vi "Open Data File.vi"(8 "error in (no error)":errorcluster, 11 "DbMeasurement in":refnum<class "DbMeasurement.lvclass">) -> (0 "error out":errorcluster, 3 "DbMeasurement out":refnum<class "DbMeasurement.lvclass">)   [LabVIEW 2013, in "DbMeasurement.lvclass"]
doc: "This static method opens the data file, which points to a database link."
uses:
  DbMeasurement.lvclass
  BaseMeasurement/BaseMeasurement.lvclass/BaseMeasurement.ctl
  DbMeasurement.lvclass/DbMeasurement.ctl
  <vilib>/addons/database/Connection.llb/DB Tools Open Connec (String).vi
  BaseMeasurement/BaseMeasurement.lvclass
  <vilib>/addons/database/NI_Database_API.lvlib
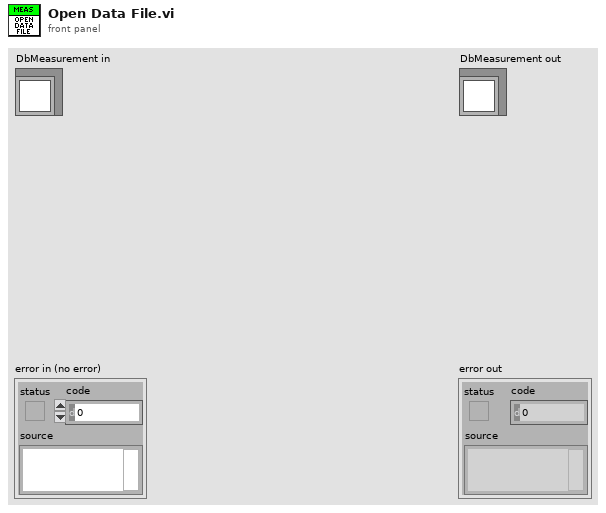
[diagram p1: front panel]
types:
  T1 = typedef "NI_Database_API.lvlib/Conn ObjectReference.ctl" = refnum<k1>
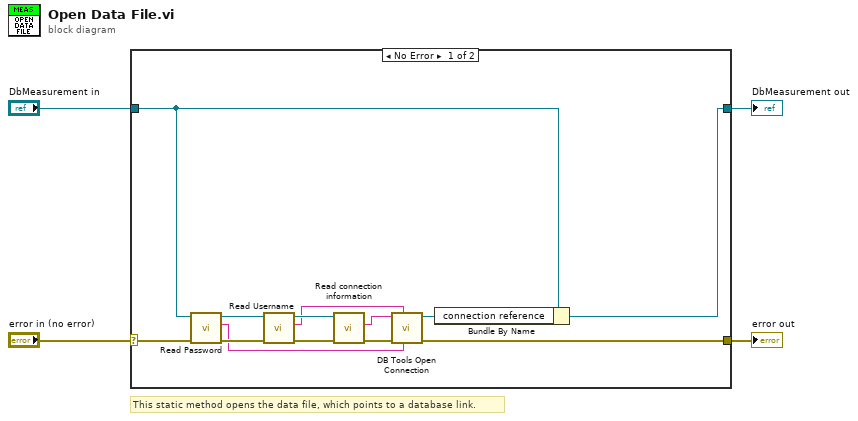
[diagram p0: block diagram]
diagram:
  # "This static method opens the data file, which points to a database link."
  n1 = case shown="No Error" "error in (no error)" {
    selector: "error in (no error)" -> [w15 w19]
    tunnel: [w5 w19] -> w3
    tunnel: [w6 w18] -> w1
    tunnel: "DbMeasurement in" -> [w12 w18]
    frame No Error {
      n2 = call "Read Password.vi"("error in (no error)"=w15, "BaseMeasurement in"=w12) -> ("error out"=w14:errorcluster, "Password"=w8:string, "BaseMeasurement out"=w11:refnum<class "DbMeasurement.lvclass">)  [unwired: 7 in]
      n3 = call "Read Username.vi"("error in (no error)"=w14, "BaseMeasurement in"=w11) -> ("error out"=w13:errorcluster, "Username"=w9:string, "BaseMeasurement out"=w10:refnum<class "DbMeasurement.lvclass">)  [unwired: 7 in]
      n4 = call "Read connection information.vi"("error in (no error)"=w13, "BaseMeasurement in"=w10) -> ("error out"=w17:errorcluster, "connection information"=w7:string)  [unwired: 7 in, 1 out]
      n5 = call-poly <vilib>:"DB Tools Open Connection.vi"("password"=w8, "userID"=w9, "error in (no error)"=w17, "connection information"=w7) -> ("error out"=w5:errorcluster, "connection reference"=w16:T1)  [unwired: 4 in]
      n6 = Bundle By Name(cluster=w12, "connection reference"=w16) -> (w6:refnum<class "DbMeasurement.lvclass">)
    }
    frame Error {
    }
  }
  "error out" <- w3
  "DbMeasurement out" <- w1
